vi "Write Available Channels.vi"(0 "IO Device in":refnum<class "IO Device.lvclass">=refnum, 1 "All Daq Channels":tag[](array[tag]), 2 "DAQ Channel Info":T1, 3 "Used DAQChannels":tag[](array[tag])) -> (7 "IO Device out":refnum<class "IO Device.lvclass">)   [LabVIEW 2015, in "IO Device.lvlib" / "IO Device.lvclass"]
uses:
  IO Device.lvclass
  Sequencer/Sequencer/Daq Channel Info.ctl
  Simulated DAQ/Simulated DAQ/Simulated DAQ.lvclass
  <vilib>/ActorFramework/Message Enqueuer/Message Enqueuer.lvclass
  <vilib>/ActorFramework/Message Priority Queue/Message Priority Queue.lvclass
  IODevInfo.lvclass
  IODevConfig.lvclass
  IO Device.lvclass/IO Device.ctl
  Read IODevInfo.vi
  Write IODevInfo.vi
  Sequencer/Sequencer/Sequencer.lvclass
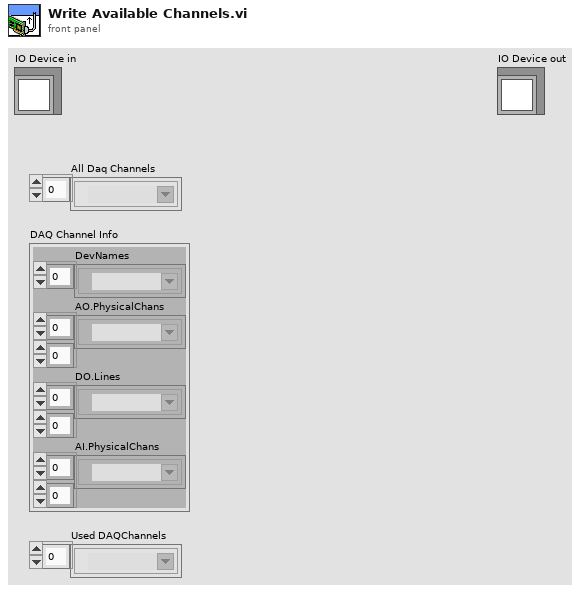
[diagram p1: front panel]
types:
  T1 = typedef "Sequencer.lvlib/Sequencer.lvclass/Daq Channel Info.ctl" = cluster{"DevNames":tag[], "AO.PhysicalChans":tag[][], "DO.Lines":tag[][], "AI.PhysicalChans":tag[][]}
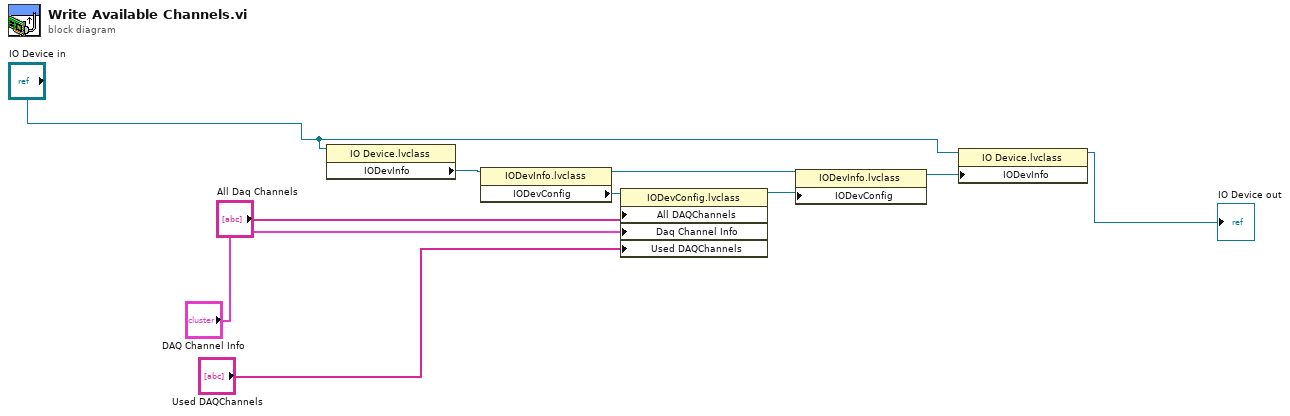
[diagram p0: block diagram]
diagram:
  n1 = property class="IO Device.lvclass"(reference="IO Device in") -> ("IODevInfo"=w6:refnum<class "IODevInfo.lvclass">)  [unwired: 1 in, 2 out]
  n2 = property class="IODevInfo.lvclass"(reference=w6) -> (reference out=w8:refnum<class "IODevInfo.lvclass">, "IODevConfig"=w7:refnum<class "IODevConfig.lvclass">)  [unwired: 1 in, 1 out]
  n3 = property class="IODevConfig.lvclass"(reference=w7, "All DAQChannels"="All Daq Channels", "Daq Channel Info"="DAQ Channel Info", "Used DAQChannels"="Used DAQChannels") -> (reference out=w9:refnum<class "IODevConfig.lvclass">)  [unwired: 1 in, 1 out]
  n4 = property class="IODevInfo.lvclass"(reference=w8, "IODevConfig"=w9) -> (reference out=w10:refnum<class "IODevInfo.lvclass">)  [unwired: 1 in, 1 out]
  n5 = property class="IO Device.lvclass"(reference="IO Device in", "IODevInfo"=w10) -> (reference out=→"IO Device out":refnum<class "IO Device.lvclass">)  [unwired: 1 in, 1 out]
